vi "Cmd Sync with OPC and SRQ - learn.vi"() -> ()   [LabVIEW 2011]
doc: "Instructs the instrument to issue a service request when the operation associated with the command is complete.\n\nUse this VI for instructional purposes. If you plan on using service requests in your application to synchronize commands using the operation complete (OPC) method, please refer to Example Command Sync using OPC and SRQ 2.vi. \n\nTo use the VI, complete the following steps: \n \n\n1. Select your instrument resource name from the VISA session drop down menu.\n\nThe registers are pre-configured for issuing a SRQ when either an instrument error occurs or when the desired operation is complete. To guarantee the behavior of this VI, it is recommended you do not modify the register controls.\n\n2. Run the VI.\n\nEach time you select the \"Send\" button, the contents of the Write Buffer are sent to the instrument. The output register indicate the values of the event registers after the wait on the service requests ends.\n\n3. Select the \"Stop\" button to terminate the VI.\n\nNote: The default commands used in this example work with the Agilent 34401A using the GPIB interface. You can use this VI with other instruments that use the IEEE 488.2 registers. However, you should read your instrument manual for specific details of the commands you send to the instrument."
uses:
  Low Level/Standadard Event Status Enable Control.ctl
  Low Level/Service Request Enable Control.ctl
  Low Level/Standard Event Status Indicator.ctl
  Low Level/Status Byte Indicator.ctl
  <vilib>/Instr/_visa.llb/Select Event Type.ctl
panel:
  out "Read SBR":T1
  out "Read SESR":T2
  in  "Enable SRER":T3={" Instrument Specific (1)"=FALSE, " Instrument Specific (2)"=FALSE, " Instrument Specific (4)"=FALSE, " Instrument Specific (8)"=FALSE, "Message Available (16)"=FALSE, "Event Status Bit (32)"=TRUE, "Request for Service (64)"=FALSE, " Instrument Specific (128)"=FALSE}
  in  "Enable SESER":T4={"Operation Complete (1)"=TRUE, "Request Control (2)"=FALSE, "Query Error (4)"=TRUE, "Device Dependent Error (8)"=TRUE, "Execution Error (16)"=TRUE, "Command Error (32)"=TRUE, "User Request (64)"=FALSE, "Power On (128)"=FALSE}
  in  "Send":bool
  in  "STOP":bool
  in  "Command":string=":TRIG:COUN 1;:INIT"
  in  "VISA session":refnum<visa-resource-name>
  # "This VI instructs the instrument to issue a service\nrequest when the operation associated with the\ncommand is complete."
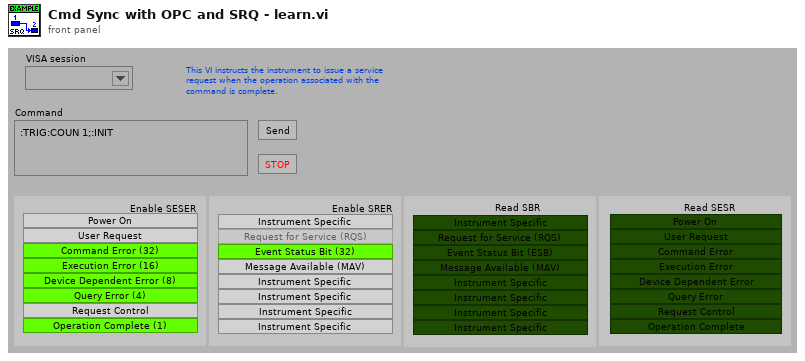
[diagram p1: front panel]
types:
  T1 = typedef "Status Byte Indicator.ctl" = cluster{"Instrument Specific (1)":bool, "Instrument Specific (2)":bool, "Instrument Specific (4)":bool, "Instrument Specific (8)":bool, "Message Available (16)":bool, "Event Status Bit (32)":bool, "Request for Service (32)":bool, "Instrument Specific (128)":bool}
  T2 = typedef "Standard Event Status Indicator.ctl" = cluster{"Operation Complete (1)":bool, "Request Control (2)":bool, "Query Error (4)":bool, "Device Dependent Error (8)":bool, "Execution Error (16)":bool, "Command Error (32)":bool, "User Request (64)":bool, "Power On (128)":bool}
  T3 = typedef "Service Request Enable Control.ctl" = cluster{" Instrument Specific (1)":bool, " Instrument Specific (2)":bool, " Instrument Specific (4)":bool, " Instrument Specific (8)":bool, "Message Available (16)":bool, "Event Status Bit (32)":bool, "Request for Service (64)":bool, " Instrument Specific (128)":bool}
  T4 = typedef "Standadard Event Status Enable Control.ctl" = cluster{"Operation Complete (1)":bool, "Request Control (2)":bool, "Query Error (4)":bool, "Device Dependent Error (8)":bool, "Execution Error (16)":bool, "Command Error (32)":bool, "User Request (64)":bool, "Power On (128)":bool}
  T5 = typedef "Select Event Type.ctl" = u32
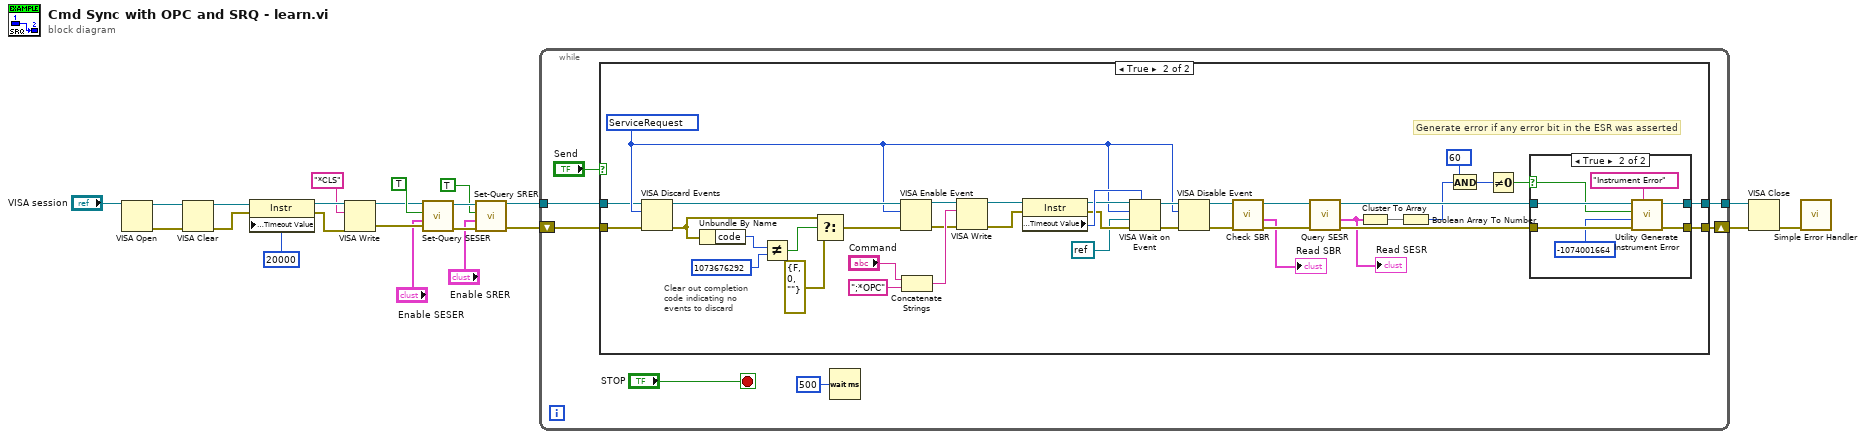
[diagram p0: block diagram]
diagram:
  n1 = VISA Open(VISA resource name="VISA session") -> (VISA resource name=w5:refnum<visa-resource-name>, error out=w4:errorcluster)  [unwired: 4 in]
  n2 = VISA Clear(VISA resource name=w5, error in (no error)=w4) -> (VISA resource name out=w3:refnum<visa-resource-name>, error out=w2:errorcluster)
  n3 = property class="Instr"(reference=w3, error in=w2, "General Settings:Timeout Value"=u32 20000) -> (reference out=w13:refnum<visa-resource-name>, error out=w12:errorcluster)
  n4 = VISA Write(VISA resource name=w13, write buffer="*CLS", error in (no error)=w12) -> (VISA resource name out=w10:refnum<visa-resource-name>, error out=w9:errorcluster)  [unwired: 1 out]
  n5 = call "Set-Query SESER.vi"("error in (no error)"=w9, "Enable SESER"="Enable SESER", "Enable Mask (T)"=TRUE ("Enable Mask"), "VISA session"=w10) -> ("error out"=w17:errorcluster, "dup VISA session"=w18:refnum<visa-resource-name>)  [unwired: 5 in, 1 out]
  n6 = call "Set-Query SRER.vi"("error   in (no error)"=w17, "Enable SRER"="Enable SRER", "Enable Mask (T)"=TRUE ("function"), "VISA session"=w18) -> ("error out"=w1:errorcluster, "dup VISA session"=w6:refnum<visa-resource-name>)  [unwired: 5 in, 1 out]
  n7 = while {
    tunnel: [w28] -> w20
    tunnel: w6 -> [w24]
    shift-right: [w29] -> w19
    shift-left: w1 -> [w23]
    stop <- "STOP" stop-if-true
    n8 = case shown="True" "Send" {
      tunnel: [w31 w61] -> w29
      tunnel: [w30 w62] -> w28
      tunnel: w23 -> [w31 w37]
      tunnel: w24 -> [w30 w41]
      frame False {
      }
      frame True {
        w42 = T5 1073684491 items=["ServiceRequest"=1073684491, "Trigger"=3221168138, "Clear"=1073684493, "VXI-Signal"=1073684512, "VXI/VME-Interrupt"=3221168161, "VXI/VME-Sysfail"=1073684509, "VXI/VME-Sysreset"=1073684510, "GPIB-CIC"=1073684498, "GPIB-Talk"=1073684499, "GPIB-Listen"=1073684500, "PXI-Interrupt"=1073684514, "AllEnabled"=1073709055] ("Event Type")
        # "Clear out completion\ncode indicating no \nevents to discard"
        # "Generate error if any error bit in the ESR was asserted"
        n9 = VISA Discard Events(8:w37, 10:w42, 11:w41) -> (0:w47:errorcluster, 3:w43:refnum<visa-resource-name>)  [unwired: 1 in]
        n10 = Unbundle By Name(w47) -> ("code"=w44:i32)
        n11 = Not Equal?(x=w44, y=1073676292 ("code")) -> (x != y?=w46:bool)
        n12 = Select(t=w47, s=w46, f=errorcluster {"status"=FALSE, "code"=0, "source"=""} ("error cluster")) -> (s? t:f=w49:errorcluster)
        n13 = VISA Enable Event(8:w49, 10:w42, 11:w43) -> (0:w54:errorcluster, 3:w53:refnum<visa-resource-name>)  [unwired: 1 in]
        n14 = Concatenate Strings("Command", ";*OPC" ("string")) -> (w59:string)
        n15 = VISA Write(VISA resource name=w53, write buffer=w59, error in (no error)=w54) -> (VISA resource name out=w51:refnum<visa-resource-name>, error out=w52:errorcluster)  [unwired: 1 out]
        n16 = property class="Instr"(reference=w51, error in=w52) -> (reference out=w55:refnum<visa-resource-name>, error out=w56:errorcluster, "General Settings:Timeout Value"=w60:u32)
        n17 = VISA Wait on Event(7:w60, 8:w56, 9:refnum<visa-resource-name> refnum ("event resource class"), 10:w42, 11:w55) -> (0:w58:errorcluster, 3:w57:refnum<visa-resource-name>)  [unwired: 2 out]
        n18 = VISA Disable Event(8:w58, 10:w42, 11:w57) -> (0:w35:errorcluster, 3:w36:refnum<visa-resource-name>)  [unwired: 1 in]
        n19 = call "Check SBR.vi"("error in (no error)"=w35, "VISA session"=w36) -> ("error out"=w33:errorcluster, "Read SBR"=→"Read SBR":T1, "dup VISA session"=w34:refnum<visa-resource-name>)  [unwired: 7 in]
        n20 = call "Query SESR.vi"("error in (no error)"=w33, "VISA session"=w34) -> ("error out"=w64:errorcluster, "Read SESR"=w38:T2, "dup VISA session"=w65:refnum<visa-resource-name>)  [unwired: 7 in]
        "Read SESR" <- w38
        n21 = Cluster To Array(cluster=w38) -> (array=w66:bool[])
        n22 = Boolean Array To Number(Boolean array=w66) -> (number=w63:u32)
        n23 = And(x=60, y=w63) -> (x .and. y?=w68:u32)
        n24 = Not Equal To 0?(x=w68) -> (x != 0?=w67:bool)
        n25 = case shown="True" w67 {
          selector: w67 -> [_ w74]
          tunnel: w65 -> [w71 w78]
          tunnel: w64 -> [w70 w77]
          tunnel: [w71 w76] -> w62
          tunnel: [w70 w75] -> w61
          frame False {
          }
          frame True {
            n26 = call "Utility Generate Instrument Error.vi"("Message"="Instrument Error", "error in (no error)"=w77, "Code (0)"=-1074001664 ("x"), "Is Warning? (F)"=w74, "VISA session"=w78) -> ("error out"=w75:errorcluster, "dup VISA session"=w76:refnum<visa-resource-name>)  [unwired: 5 in]
          }
        }
      }
    }
    n27 = Wait (ms)(milliseconds to wait=u32 500) -> ()  [unwired: 1 out]
  }
  n28 = VISA Close(VISA resource name=w20, error in (no error)=w19) -> (error out=w8:errorcluster)
  n29 = call <vilib>:"Simple Error Handler.vi"("error in (no error)"=w8) -> ()  [unwired: 4 in, 5 out]
